vi "Get Source File Paths.vi"(0 "serial output channels":string[](array[string]), 5 "base tdms file path":path) -> (4 "source file paths":T1[](array[typedef]))   [LabVIEW 2023, in "GettingStarted_Gen_148X_Host.lvlib"]
uses:
  GettingStarted_Gen_148X_Host.lvlib
  Types/Channel Source File Paths.ctl
  <instrlib>/FlexRIO/Automotive Vision Utility/v1/Host/Automotive Vision Utility.lvlib
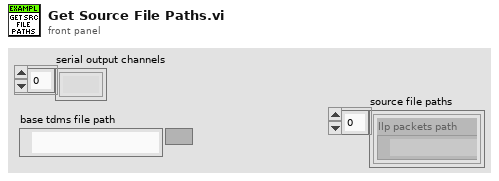
[diagram p1: front panel]
types:
  T1 = typedef "GettingStarted_Gen_148X_Host.lvlib/Channel Source File Paths.ctl" = cluster{"llp packets path":path}
  T2 = typedef "Automotive Vision Utility.lvlib/Serial Channel Type.ctl" = enum16{"Serial Input Channel", "Serial Output Channel", "Unknown Channel Type"}
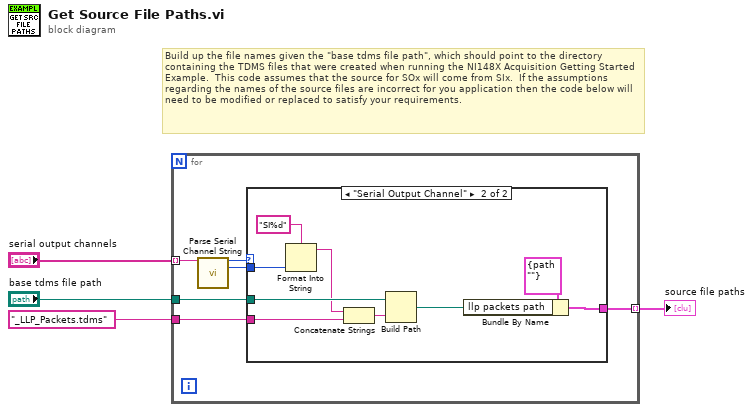
[diagram p0: block diagram]
diagram:
  # "Build up the file names given the \"base tdms file path\", which should point to the directory containing the TDMS files that were created when running the NI148X Acquisition Getting Started Example.  This code assumes that the source for SOx will come from SIx.  If the assumptions regarding the names of the source files are incorrect for you application then the code below will need to be modified or replaced to satisfy your requirements."
  n1 = for {
    tunnel: "serial output channels" -> [w8] mode=indexing
    tunnel: "base tdms file path" -> [w10]
    tunnel: "_LLP_Packets.tdms" -> [w9]
    tunnel: [w5] -> w1 mode=indexing
    n2 = call <instrlib>:"Parse Serial Channel String.vi"("serial channel string"=w8) -> ("serial channel type"=w7:T2, "channel number"=w6:i32)  [unwired: 13 in]
    n3 = case shown="\"Serial Output Channel\"" w7 {
      tunnel: w10 -> [_ w16]
      tunnel: w9 -> [_ w15]
      tunnel: w6 -> [_ w13]
      tunnel: [_ w11] -> w5
      frame "Serial Input Channel", Default {
      }
      frame "Serial Output Channel" {
        n4 = Format Into String(format string="SI%d", w13) -> (resulting string=w12:string)  [unwired: 2 in, 1 out]
        n5 = Concatenate Strings(w12, w15) -> (w19:string)
        n6 = Build Path(base path=w16, name or relative path=w19) -> (appended path=w17:path)
        n7 = Bundle By Name(cluster=T1 {"llp packets path"=path ""} ("channel source file paths"), "llp packets path"=w17) -> (w11:T1)
      }
    }
  }
  "source file paths" <- w1
